vi "生成报告.vi"(0 "打印?":bool, 2 "输出簇":T1) -> ()   [LabVIEW 2010]
uses:
  <vilib>/Utility/NIReport.llb/Append Report Text (str wrap).vi
  <vilib>/addons/_office/word.llb/Word Easy Table (str).vi
  <vilib>/Utility/NIReport.llb/NI_report.lvclass
  <vilib>/addons/_office/NI_ReportGenerationToolkit.lvlib
panel:
  in  "序号":i32
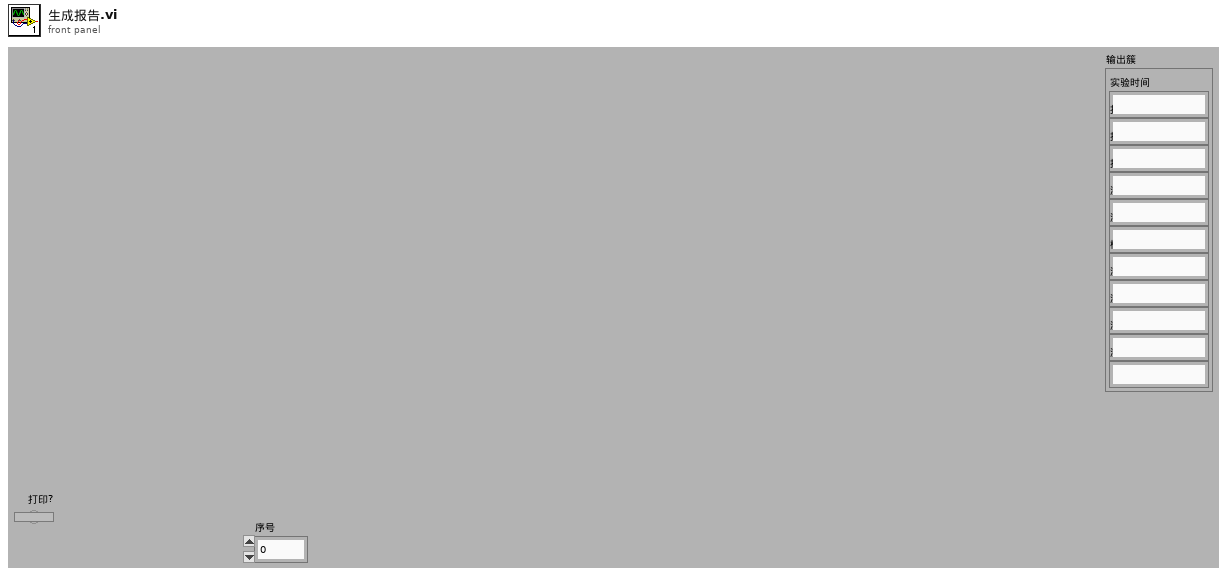
[diagram p1: front panel]
types:
  T1 = cluster{"实验时间":string, "报告编号":string, "控制板编号":string, "控制板类型":string, "测试人员":string, "测试地点":string, "概述":string, "测试项 1":string, "测试项 2":string, "测试项 3":string, "测试项 4":string}
  T2 = cluster{"position (Excel)":cluster{"row":i32, "column":i32}, "name (Excel)":string, "bookmark (Word)":string}
  T3 = enum16{"maximized", "minimized", "normal", "no change"}
  T4 = enum16{"Standard Report", "HTML", "Word", "Excel"}
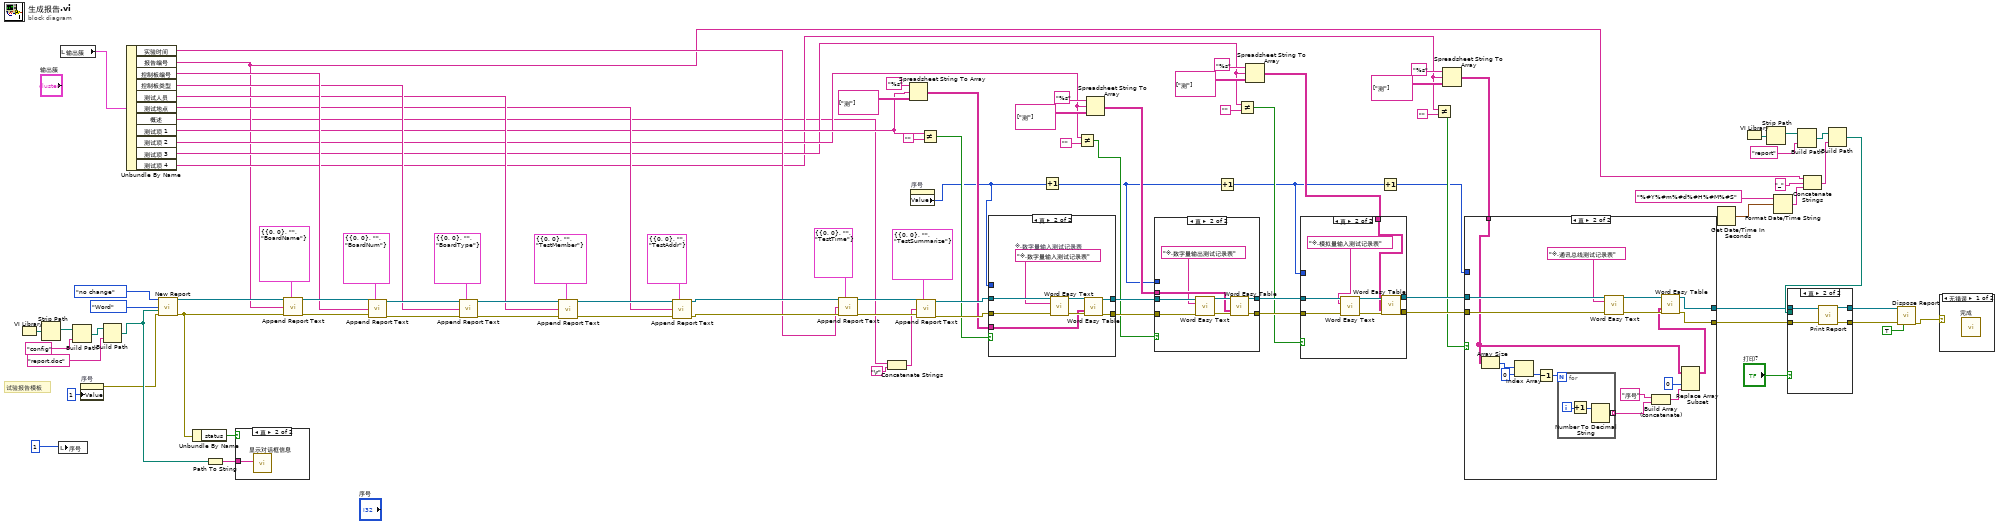
[diagram p0: block diagram]
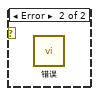
[diagram p6: hidden frame]
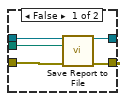
[diagram p7: hidden frame]
diagram:
  # "试验报告模板"
  n1 = VI Library() -> (path=w91:path)
  n2 = Strip Path(path=w91) -> (stripped path=w88:path)  [unwired: 1 out]
  n3 = local write "序号"(1) -> ()
  n4 = local read "输出簇"() -> (w97:T1)
  n5 = Build Path(base path=w88, name or relative path="config") -> (appended path=w90:path)
  n6 = property on="序号" class="DigNum (严格)"("Value"=1 ("序号")) -> (error out=w42:errorcluster)  [unwired: 2 in, 1 out]
  n7 = Build Path(base path=w90, name or relative path="report.doc") -> (appended path=w94:path)
  n8 = Unbundle By Name(w97) -> ("实验时间"=w34:string, "报告编号"=w8:string, "控制板编号"=w38:string, "控制板类型"=w37:string, "测试人员"=w36:string, "测试地点"=w35:string, "概述"=w7:string, "测试项 1"=w29:string, "测试项 2"=w24:string, "测试项 3"=w18:string, "测试项 4"=w12:string)
  n9 = call <vilib>:"New Report.vi"("window state (normal)"=T3."no change", "report type"=T4."Word", "template (empty)"=w94, "error in (no error)"=w42) -> ("report out"=w85:refnum<class "NI_report.lvclass">, "error out"=w84:errorcluster)  [unwired: 10 in]
  n10 = Unbundle By Name(w84) -> ("status"=w96:bool)
  n11 = Path To String(path=w94) -> (string=w95:string)
  n12 = case shown="真" w96 {
    tunnel: w95 -> [_ w98]
    frame False {
    }
    frame True {
      n13 = call "显示对话框信息"("Message"=w98) -> ()  [unwired: 9 in, 2 out]
    }
  }
  n14 = call-poly <vilib>:"Append Report Text.vi"("report in"=w85, "MS Office parameters"=T2 {"position (Excel)"={"row"=0, "column"=0}, "name (Excel)"="", "bookmark (Word)"="BoardName"}, "text"=w8, "error in (no error)"=w84) -> ("report out"=w70:refnum<class "NI_report.lvclass">, "error out"=w69:errorcluster)  [unwired: 8 in, 2 out]
  n15 = call-poly <vilib>:"Append Report Text.vi"("report in"=w70, "MS Office parameters"=T2 {"position (Excel)"={"row"=0, "column"=0}, "name (Excel)"="", "bookmark (Word)"="BoardNum"}, "text"=w38, "error in (no error)"=w69) -> ("report out"=w80:refnum<class "NI_report.lvclass">, "error out"=w79:errorcluster)  [unwired: 8 in, 2 out]
  n16 = call-poly <vilib>:"Append Report Text.vi"("report in"=w80, "MS Office parameters"=T2 {"position (Excel)"={"row"=0, "column"=0}, "name (Excel)"="", "bookmark (Word)"="BoardType"}, "text"=w37, "error in (no error)"=w79) -> ("report out"=w77:refnum<class "NI_report.lvclass">, "error out"=w76:errorcluster)  [unwired: 8 in, 2 out]
  n17 = call-poly <vilib>:"Append Report Text.vi"("report in"=w77, "MS Office parameters"=T2 {"position (Excel)"={"row"=0, "column"=0}, "name (Excel)"="", "bookmark (Word)"="TestMember"}, "text"=w36, "error in (no error)"=w76) -> ("report out"=w74:refnum<class "NI_report.lvclass">, "error out"=w73:errorcluster)  [unwired: 8 in, 2 out]
  n18 = call-poly <vilib>:"Append Report Text.vi"("report in"=w74, "MS Office parameters"=T2 {"position (Excel)"={"row"=0, "column"=0}, "name (Excel)"="", "bookmark (Word)"="TestAddr"}, "text"=w35, "error in (no error)"=w73) -> ("report out"=w72:refnum<class "NI_report.lvclass">, "error out"=w71:errorcluster)  [unwired: 8 in, 2 out]
  n19 = call-poly <vilib>:"Append Report Text.vi"("report in"=w72, "MS Office parameters"=T2 {"position (Excel)"={"row"=0, "column"=0}, "name (Excel)"="", "bookmark (Word)"="TestTime"}, "text"=w34, "error in (no error)"=w71) -> ("report out"=w47:refnum<class "NI_report.lvclass">, "error out"=w46:errorcluster)  [unwired: 8 in, 2 out]
  n20 = Concatenate Strings(w7, "\r") -> (w5:string)
  n21 = Spreadsheet String To Array(format string="%s" ("格式字符串"), spreadsheet string=w29, array type (2D Dbl)=string[][] [["测"]] ("数组类型(2D String)")) -> (array=w28:string[][])  [unwired: 1 in]
  n22 = property on="序号" class="DigNum (严格)"() -> ("Value"=w4:i32)  [unwired: 2 in, 2 out]
  n23 = call-poly <vilib>:"Append Report Text.vi"("report in"=w47, "MS Office parameters"=T2 {"position (Excel)"={"row"=0, "column"=0}, "name (Excel)"="", "bookmark (Word)"="TestSummarize"}, "text"=w5, "error in (no error)"=w46) -> ("report out"=w45:refnum<class "NI_report.lvclass">, "error out"=w44:errorcluster)  [unwired: 8 in, 2 out]
  n24 = Not Equal?(x=w29, y="") -> (x != y?=w32:bool)
  n25 = case shown="真" w32 {
    tunnel: [w100 w107] -> w54
    tunnel: [w99 w106] -> w52
    tunnel: w45 -> [w100 w104]
    tunnel: w44 -> [w99 w103]
    tunnel: w4 -> [_ _]
    tunnel: w28 -> [_ w102]
    frame False {
    }
    frame True {
      w101 = "※.数字量输入测试记录表"  # ※.数字量输入测试记录表
      n26 = call <vilib>:"Word Easy Text.vi"("report in"=w104, "text"=w101, "error in (no error)"=w103) -> ("report out"=w108:refnum<class "NI_report.lvclass">, "error out"=w105:errorcluster)  [unwired: 10 in, 1 out]
      n27 = call-poly <vilib>:"Word Easy Table.vi"("report in"=w108, "data"=w102, "error in (no error)"=w105) -> ("report out"=w107:refnum<class "NI_report.lvclass">, "error out"=w106:errorcluster)  [unwired: 10 in, 1 out]
    }
  }
  n28 = Increment(x=w4) -> (x+1=w3:i32)
  n29 = Not Equal?(x=w24, y="") -> (x != y?=w23:bool)
  n30 = Spreadsheet String To Array(format string="%s" ("格式字符串"), spreadsheet string=w24, array type (2D Dbl)=string[][] [["测"]] ("数组类型(2D String)")) -> (array=w22:string[][])  [unwired: 1 in]
  n31 = case shown="真" w23 {
    tunnel: w54 -> [w110 w118]
    tunnel: [w110 w116] -> w53
    tunnel: w52 -> [w109 w115]
    tunnel: [w109 w113] -> w51
    tunnel: w3 -> [_ _]
    tunnel: w22 -> [_ w112]
    frame False {
    }
    frame True {
      n32 = call <vilib>:"Word Easy Text.vi"("report in"=w118, "text"="※.数字量输出测试记录表", "error in (no error)"=w115) -> ("report out"=w117:refnum<class "NI_report.lvclass">, "error out"=w114:errorcluster)  [unwired: 10 in, 1 out]
      n33 = call-poly <vilib>:"Word Easy Table.vi"("report in"=w117, "data"=w112, "error in (no error)"=w114) -> ("report out"=w116:refnum<class "NI_report.lvclass">, "error out"=w113:errorcluster)  [unwired: 10 in, 1 out]
    }
  }
  n34 = Increment(x=w3) -> (x+1=w2:i32)
  n35 = Not Equal?(x=w18, y="") -> (x != y?=w17:bool)
  n36 = Spreadsheet String To Array(format string="%s" ("格式字符串"), spreadsheet string=w18, array type (2D Dbl)=string[][] [["测"]] ("数组类型(2D String)")) -> (array=w16:string[][])  [unwired: 1 in]
  n37 = case shown="真" w17 {
    tunnel: w53 -> [w120 w128]
    tunnel: w51 -> [w119 w126]
    tunnel: [w120 w124] -> w50
    tunnel: [w119 w123] -> w49
    tunnel: w2 -> [_ _]
    tunnel: w16 -> [_ w122]
    frame False {
    }
    frame True {
      n38 = call <vilib>:"Word Easy Text.vi"("report in"=w128, "text"="※.模拟量输入测试记录表", "error in (no error)"=w126) -> ("report out"=w127:refnum<class "NI_report.lvclass">, "error out"=w125:errorcluster)  [unwired: 10 in, 1 out]
      n39 = call-poly <vilib>:"Word Easy Table.vi"("report in"=w127, "data"=w122, "error in (no error)"=w125) -> ("report out"=w124:refnum<class "NI_report.lvclass">, "error out"=w123:errorcluster)  [unwired: 10 in, 1 out]
    }
  }
  n40 = Increment(x=w2) -> (x+1=w1:i32)
  n41 = Not Equal?(x=w12, y="") -> (x != y?=w11:bool)
  n42 = Spreadsheet String To Array(format string="%s" ("格式字符串"), spreadsheet string=w12, array type (2D Dbl)=string[][] [["测"]] ("数组类型(2D String)")) -> (array=w10:string[][])  [unwired: 1 in]
  n43 = case shown="真" w11 {
    tunnel: [w130 w147] -> w56
    tunnel: [w129 w146] -> w55
    tunnel: w50 -> [w130 w145]
    tunnel: w49 -> [w129 w144]
    tunnel: w1 -> [_ _]
    tunnel: w10 -> [_ w132]
    frame False {
    }
    frame True {
      n44 = Array Size(array=w132) -> (size(s)=w133:i32[])
      n45 = Index Array(array=w133, index=0 ("索引")) -> (element=w136:i32)
      n46 = Decrement(x=w136) -> (x-1=w137:i32)
      n47 = for {
        N: w137 -> [_]
        tunnel: [w148] -> w139 mode=indexing
        i -> [w150]
        n48 = Increment(x=w150) -> (x+1=w149:i32)
        n49 = Number To Decimal String(number=w149) -> (decimal integer string=w148:string)  [unwired: 1 in]
      }
      n50 = call <vilib>:"Word Easy Text.vi"("report in"=w145, "text"="※.通讯总线测试记录表", "error in (no error)"=w144) -> ("report out"=w143:refnum<class "NI_report.lvclass">, "error out"=w142:errorcluster)  [unwired: 10 in, 1 out]
      n51 = Build Array (concatenate)("序号", w139) -> (w140:string[])
      n52 = Replace Array Subset(array=w132, new element=w140, index (col)=0 ("索引 (行)")) -> (w131:string[][])  [unwired: 1 in]
      n53 = call-poly <vilib>:"Word Easy Table.vi"("report in"=w143, "data"=w131, "error in (no error)"=w142) -> ("report out"=w147:refnum<class "NI_report.lvclass">, "error out"=w146:errorcluster)  [unwired: 10 in, 1 out]
    }
  }
  n54 = Get Date/Time In Seconds() -> (seconds since 1Jan1904=w63:timestamp)
  n55 = VI Library() -> (path=w64:path)
  n56 = Strip Path(path=w64) -> (stripped path=w67:path)  [unwired: 1 out]
  n57 = Format Date/Time String(time format string (%c)="%#Y%#m%#d%#H%#M%#S" ("时间格式字符串(%c)"), seconds (now)=w63) -> (date/time string=w41:string)  [unwired: 1 in]
  n58 = Build Path(base path=w67, name or relative path="report") -> (appended path=w65:path)
  n59 = Concatenate Strings(w8, "_", w41) -> (w39:string)
  n60 = Build Path(base path=w65, name or relative path=w39) -> (appended path=w58:path)
  n61 = case shown="真" "打印?" {
    tunnel: w56 -> [w155 w159]
    tunnel: w55 -> [w154 w158]
    tunnel: [w153 w157] -> w61
    tunnel: [w152 w156] -> w60
    tunnel: w58 -> [w151 _]
    frame False {
      n62 = call-dynamic "Save Report to File.vi"("report in"=w155, "report file path"=w151, "error in (no error)"=w154) -> ("report out"=w153:refnum<class "NI_report.lvclass">, "error out"=w152:errorcluster)  [unwired: 11 in]
    }
    frame True {
      n63 = call-dynamic "Print Report.vi"("report in"=w159, "error in (no error)"=w158) -> ("report out"=w157:refnum<class "NI_report.lvclass">, "error out"=w156:errorcluster)  [unwired: 12 in]
    }
  }
  n64 = call-dynamic "Dispose Report.vi"("report in"=w61, "error in (no error)"=w60, "close report? (T)"=TRUE) -> ("error out"=w57:errorcluster)  [unwired: 12 in]
  n65 = case shown="无错误" w57 {
    frame No Error {
      n66 = call "完成"() -> ()  [unwired: 10 in, 2 out]
    }
    frame Error {
      n67 = call "错误"() -> ()  [unwired: 10 in, 2 out]
    }
  }
